vi "DMM Measurement.vi"() -> ()   [LabVIEW 2021]
doc: "This example acquires a single measurement from a National Instruments DMM. Select the measurement function and range. Specify the resolution in digits of precision. The measured value will be displayed in the Measurement indicator. The Boolean indicator will indicate if the measured value is out of range."
uses:
  <instrlib>/niDMM/nidmm.llb/niDMM Configure Measurement Digits.vi
  <instrlib>/niDigital/niDigital.llb/niDigital Selected Function.ctl
  <instrlib>/niDigital/niDigital.llb/niDigital Get Site Results Site Numbers.vi
  <instrlib>/niDigital/niDigital.llb/niDigital Burst Pattern (Pass Fail).vi
  <instrlib>/niDMM/nidmm.llb/niDMM Function.ctl
  <instrlib>/niDMM/nidmm.llb/niDMM Resolution in Digits.ctl
panel:
  in  "Digital Pattern":refnum<k15>="PXI1Slot2,PXI1Slot3" caption="resource name"
  in  "Simulate?":bool=TRUE
  out "Pass?":bool[](array[boolean])
  out "Site":string[](array[string])
  out "error out":errorcluster
  in  "error in":errorcluster caption="error in (no error)"
  in  "Resolution in Digits":T1=5.5 items=["3 1/2"=3.5, "4 1/2"=4.5, "5 1/2"=5.5, "6 1/2"=6.5, "7 1/2"=7.5]
  out "Absolute Resolution":dbl format="%#_3p"
  in  "Measurement Type":T2
  out "Signal Out of Range":bool
  in  "Range":dbl=10.0 format="%.2f"
  in  "Device Name":refnum<k15>="Dev1"
  out "Measurement":dbl format="%.6p"
  # "Configuration"
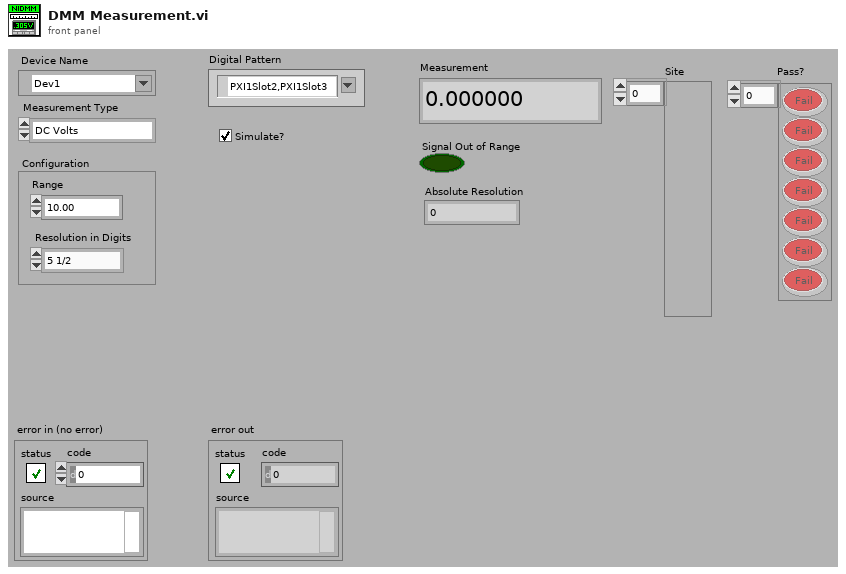
[diagram p1: front panel]
types:
  T1 = typedef "niDMM Resolution in Digits.ctl" = dbl
  T2 = typedef "niDMM Function.ctl" = enum16{"DC Volts", "AC Volts", "DC Current", "AC Current", "2-wire Resistance", "4-wire Resistance", "Diode", "Frequency", "Period", "AC Volts DC Coupled", "Capacitance", "Inductance", "Temperature"}
  T3 = typedef "niDigital Selected Function.ctl" = i32
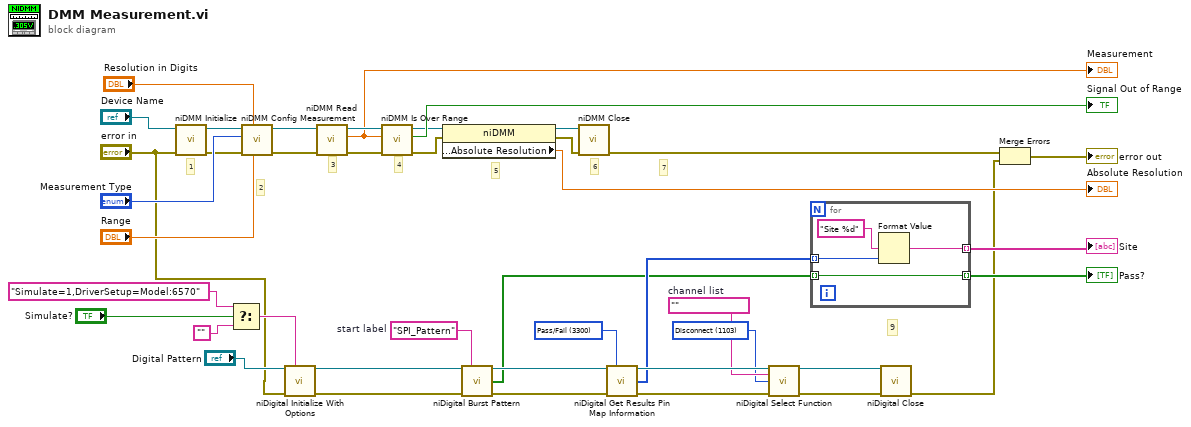
[diagram p0: block diagram]
diagram:
  w11 = ""  # channel list
  w10 = T3 1103 items=["Digital"=1100, "PPMU"=1101, "Off"=1102, "Disconnect"=1103] ("function")
  w5 = "SPI_Pattern"  # start label
  w9 = 3300 items=["Pass/Fail"=3300, "Capture Waveform"=3301] ("site result type")
  # "9"
  # "2"
  # "1"
  # "7"
  # "6"
  # "5"
  # "4"
  # "3"
  n1 = call <instrlib>:"niDMM Initialize.vi"("error in (no error)"="error in", "Instrument Descriptor"="Device Name") -> ("error out"=w33:errorcluster, "instrument handle out"=w32:refnum<k15>)  [unwired: 8 in]
  n2 = Select(t="Simulate=1,DriverSetup=Model:6570", s="Simulate?", f="") -> (s? t:f=w18:string)
  n3 = call-poly <instrlib>:"niDMM Config Measurement.vi"("Range"="Range", "Resolution in Digits"="Resolution in Digits", "error in (no error)"=w33, "Function"="Measurement Type", "instrument handle"=w32) -> ("error out"=w40:errorcluster, "instrument handle out"=w39:refnum<k15>)  [unwired: 5 in]
  n4 = call <instrlib>:"niDigital Initialize With Options.vi"("resource name"="Digital Pattern", "option string"=w18, "error in"="error in") -> ("instrument handle"=w21:refnum<k15>, "error out"=w22:errorcluster)  [unwired: 11 in]
  n5 = call <instrlib>:"niDMM Read.vi"("error in (no error)"=w40, "instrument handle"=w39) -> ("error out"=w37:errorcluster, "Measurement"=w35:dbl, "instrument handle out"=w38:refnum<k15>)  [unwired: 7 in]
  "Measurement" <- w35
  n6 = call <instrlib>:"niDMM Is Over Range.vi"("error in (no error)"=w37, "Measurement"=w35, "instrument handle"=w38) -> ("error out"=w29:errorcluster, "Over Range?"=→"Signal Out of Range":bool, "instrument handle out"=w31:refnum<k15>)  [unwired: 6 in]
  n7 = property class="niDMM"(reference=w31, error in=w29) -> (reference out=w30:refnum<k15>, error out=w28:errorcluster, "Configuration:Absolute Resolution"=→"Absolute Resolution":dbl)
  n8 = call-poly <instrlib>:"niDigital Burst Pattern.vi"("instrument handle"=w21, "start label"=w5, "error in"=w22) -> ("instrument handle out"=w6:refnum<k15>, "pass"=w4:bool[], "error out"=w7:errorcluster)  [unwired: 10 in]
  n9 = call <instrlib>:"niDMM Close.vi"("error in (no error)"=w28, "instrument handle"=w30) -> ("error out"=w25:errorcluster)  [unwired: 9 in]
  n10 = call-poly <instrlib>:"niDigital Get Results Pin Map Information.vi"("instrument handle"=w6, "site result type"=w9, "error in"=w7) -> ("instrument handle out"=w12:refnum<k15>, "site numbers"=w8:i32[], "error out"=w13:errorcluster)  [unwired: 10 in]
  n11 = call <instrlib>:"niDigital Select Function.vi"("instrument handle"=w12, "channel list"=w11, "function"=w10, "error in"=w13) -> ("instrument handle out"=w15:refnum<k15>, "error out"=w14:errorcluster)  [unwired: 10 in]
  n12 = for {
    tunnel: w4 -> [w43] mode=indexing
    tunnel: w8 -> [w45] mode=indexing
    tunnel: [w44] -> w23 mode=indexing
    tunnel: [w43] -> w24 mode=indexing
    n13 = Format Value(format string="Site %d", value (0)=w45) -> (output string=w44:string)  [unwired: 1 in]
  }
  "Pass?" <- w24
  "Site" <- w23
  n14 = call <instrlib>:"niDigital Close.vi"("instrument handle"=w15, "error in"=w14) -> ("error out"=w1:errorcluster)  [unwired: 13 in]
  n15 = Merge Errors(w25, w1) -> (→"error out":errorcluster)
